vi "Programar_Amplitud_PulsoJAVI.vi"(8 "error in (no error)":errorcluster, 10 "Numeric":dbl, 11 "VISA Refnum in":refnum<visa-resource-name>) -> (0 "Error OUT":errorcluster, 3 "VISA resource name out":refnum<visa-resource-name>="USB0::0x0957::0x4108::MY51400415::INSTR")   [LabVIEW 2019]
uses:
  Viejos/Alfredo LABVIEW/Set-up verificador ASICs/Lib Agilent 81160A/Agilent 81150/Agilent 81150.lvlib
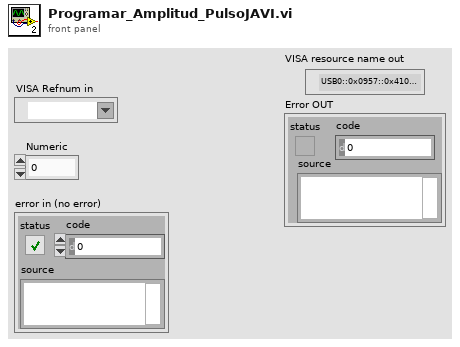
[diagram p1: front panel]
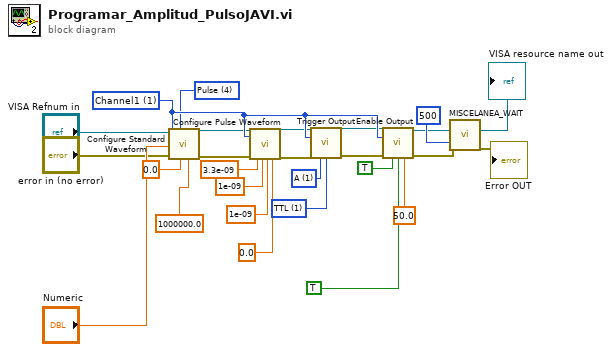
[diagram p0: block diagram]
diagram:
  w21 = u16 1 items=["ECL", "TTL"] ("Trigger Level Sync (0: ECL)")
  w20 = u16 1 items=["AB"=3, "B"=2, "A"=1, "None"=0] ("Trigger Sync Out (1: A)")
  w22 = u16 1 items=["Channel1"=1, "Channel2"=2] ("Channel (1: Channel1)")
  w13 = u16 4 items=["Sine", "Square", "Ramp Up", "Ramp Down", "Pulse", "Noise", "DC"] ("Waveform (0: Sine)")
  n1 = call "Configure Standard Waveform.vi"("Frequency (1000.0 Hz)"=1000000.0, "DC Offset (0.0 Volts)"=0.0, "Waveform (0: Sine)"=w13, "error in (no error)"="error in (no error)", "Amplitude (1.0 Vpp)"="Numeric", "Channel (1: Channel1)"=w22, "VISA resource name"="VISA Refnum in") -> ("error out"=w11:errorcluster, "VISA resource name out"=w12:refnum<visa-resource-name>)  [unwired: 3 in]
  n2 = call "Configure Pulse Waveform.vi"("VISA resource name"=w12, "Channel (1: Channel1)"=w22, "error in (no error)"=w11, "Width (1.5E-9 Sec)"=3.3e-09, "Leading Edge Time\n(1.0E-9 Sec)"=1e-09 ("Leading Edge Time\n(1.0E-9 Sec)"), "Trailing Edge Time\n(1.0E-9 Sec)"=1e-09 ("Trailing Edge Time\n(1.0E-9 Sec)"), "Delay\n(0.0 Seconds)"=0.0 ("Delay\n(0.0 Seconds)")) -> ("VISA resource name out"=w10:refnum<visa-resource-name>, "error out"=w9:errorcluster)  [unwired: 11 in]
  n3 = call "Trigger Output.vi"("VISA resource name"=w10, "Channel (1: Channel1)"=w22, "error in (no error)"=w9, "Trigger Sync Out (1: A)"=w20, "Trigger Level Sync (0: ECL)"=w21) -> ("VISA resource name out"=w8:refnum<visa-resource-name>, "error out"=w7:errorcluster)  [unwired: 9 in]
  n4 = call "Enable Output.vi"("VISA resource name"=w8, "Channel (1: Channel1)"=w22, "error in (no error)"=w7, "Enable Output (T: Enable)"=TRUE, "Enable Output Complement (T: Enable)"=TRUE, "Load (50 Ohm)"=50.0) -> ("VISA resource name out"=→"VISA resource name out":refnum<visa-resource-name>, "error out"=w6:errorcluster)  [unwired: 8 in]
  n5 = call "MISCELANEA_WAIT.vi"("ms wait IN"=u32 500, "Error IN"=w6) -> ("Error OUT"=→"Error OUT":errorcluster)  [unwired: 16 in, 1 out]
